vi "Get Table Column Headers.vi"(7 "Sheet Name":string, 8 "error in":errorcluster, 10 "Table Name":string, 11 "SpreadsheetDoc in":refnum<k24>) -> (0 "error out":errorcluster, 2 "Headers":string[](array[string]), 3 "SpreadsheetDoc out":refnum<k24>, 5 "Sheet Name":string)   [LabVIEW 2019, in "Open Xml.lvlib"]
uses:
  Open Xml.lvlib
  D:/git/Open-Xml-LabVIEW/Source/DocumentFormat.OpenXml.dll
  DocumentFormat.OpenXml.dll
  D:/git/Open-Xml-LabVIEW/Source/DocumentFormat.OpenXml.Framework.dll
  DocumentFormat.OpenXml.Framework.dll
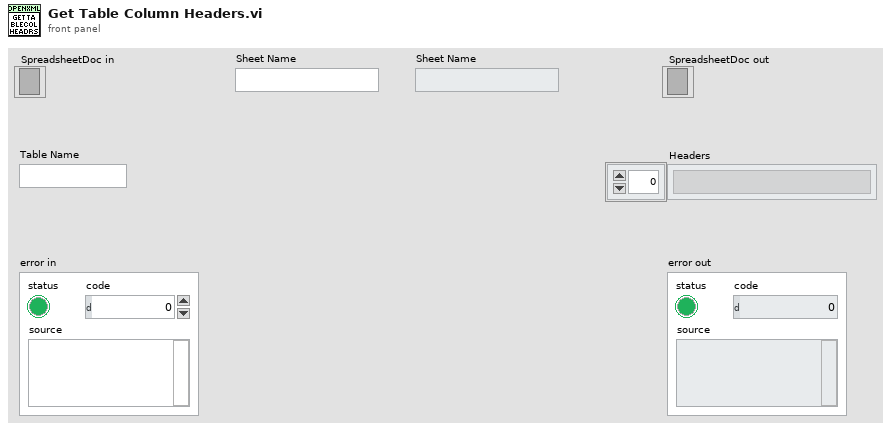
[diagram p1: front panel]
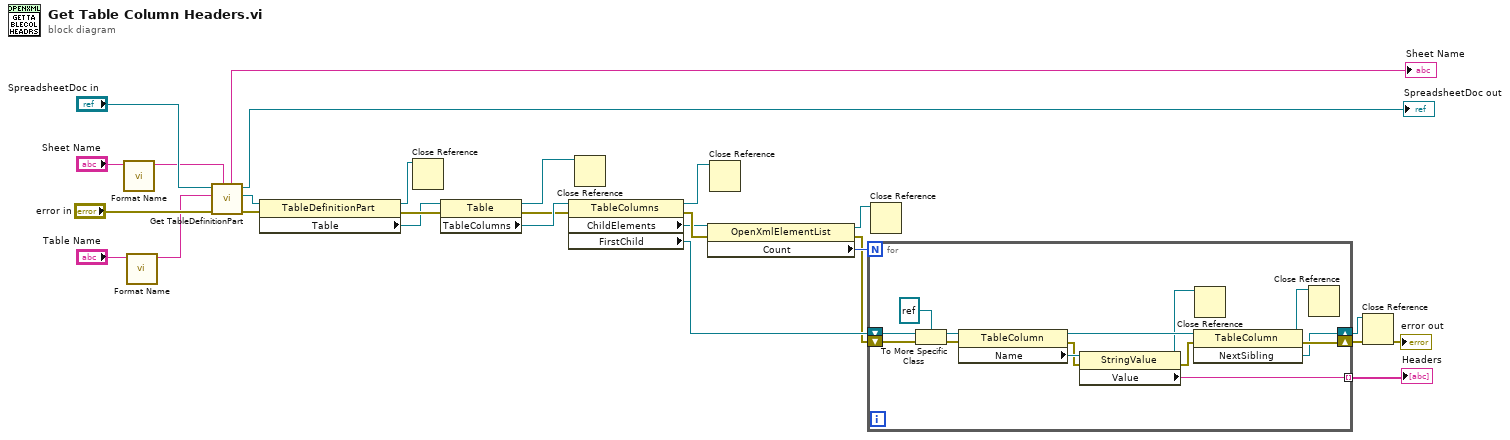
[diagram p0: block diagram]
diagram:
  n1 = call "Format Name.vi"("Sheet Name"="Sheet Name") -> ("Formatted Sheet Name"=w2:string)  [unwired: 10 in]
  n2 = call "Format Name.vi"("Sheet Name"="Table Name") -> ("Formatted Sheet Name"=w1:string)  [unwired: 10 in]
  n3 = call "Get TableDefinitionPart.vi"("Sheet Name"=w2, "error in"="error in", "Table Name"=w1, "SpreadsheetDoc in"="SpreadsheetDoc in") -> ("error out"=w16:errorcluster, "TableDefinitionPart"=w22:refnum<k24>, "SpreadsheetDo out"=→"SpreadsheetDoc out":refnum<k24>, "Sheet Name"=→"Sheet Name":string)  [unwired: 4 in]
  n4 = property class="TableDefinitionPart"(reference=w22, error in=w16) -> (reference out=w21:refnum<k24>, error out=w20:errorcluster, "Table"=w19:refnum<k24>)
  n5 = Close Reference(reference=w21) -> ()  [unwired: 1 in, 1 out]
  n6 = property class="Table"(reference=w19, error in=w20) -> (reference out=w17:refnum<k24>, error out=w6:errorcluster, "TableColumns"=w15:refnum<k24>)
  n7 = property class="TableColumns"(reference=w15, error in=w6) -> (reference out=w5:refnum<k24>, error out=w14:errorcluster, "ChildElements"=w11:refnum<k24>, "FirstChild"=w10:refnum<k24>)
  n8 = Close Reference(reference=w17) -> ()  [unwired: 1 in, 1 out]
  n9 = property class="OpenXmlElementList"(reference=w11, error in=w14) -> (reference out=w12:refnum<k24>, error out=w9:errorcluster, "Count"=w13:i32)
  n10 = Close Reference(reference=w5) -> ()  [unwired: 1 in, 1 out]
  n11 = for {
    N: w13 -> [_]
    tunnel: [w35] -> w8 mode=indexing
    shift-right: [w30] -> w3
    shift-left: w10 -> [w41]
    shift-right: [w31] -> w7
    shift-left: w9 -> [w38]
    n12 = To More Specific Class(target class=refnum<k24> refnum, reference=w41, error in=w38) -> (specific class reference=w40:refnum<k24>, error out=w37:errorcluster)
    n13 = property class="TableColumn"(reference=w40, error in=w37) -> (reference out=w34:refnum<k24>, error out=w32:errorcluster, "Name"=w36:refnum<k24>)
    n14 = property class="StringValue"(reference=w36, error in=w32) -> (reference out=w28:refnum<k24>, error out=w33:errorcluster, "Value"=w35:string)
    n15 = invoke class="TableColumn" method="NextSibling"(reference=w34, error in=w33) -> (reference out=w29:refnum<k24>, error out=w31:errorcluster, "NextSibling"=w30:refnum<k24>)  [unwired: 1 in]
    n16 = Close Reference(reference=w28) -> ()  [unwired: 1 in, 1 out]
    n17 = Close Reference(reference=w29) -> ()  [unwired: 1 in, 1 out]
  }
  "Headers" <- w8
  n18 = Close Reference(reference=w12) -> ()  [unwired: 1 in, 1 out]
  n19 = Close Reference(reference=w3, error in (no error)=w7) -> (error out=→"error out":errorcluster)
